vi "FTW-Container-FromVariant.vi"(0 "Variant":variant, 11 "error in":errorcluster) -> (4 "Name":string, 6 "Container":variant, 15 "error out":errorcluster)   [LabVIEW 2015, in "FTW-Container.lvclass"]
uses:
  FTW-Container.lvclass
  <vilib>/Utility/Data Type/NI_Data Type.lvlib
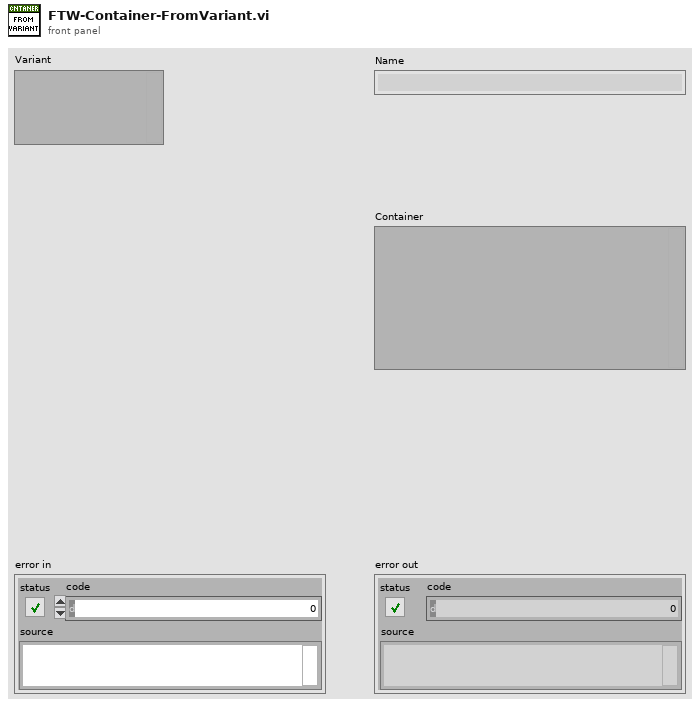
[diagram p1: front panel]
types:
  T1 = typedef "NI_Data Type.lvlib/Data Type.ctl" = enum8{"Invalid Type", "Void", "I8", "I16", "I32", "I64", "U8", "U16", "U32", "U64", "Single Float", "Double Float", "Extended Float", "Single Complex", "Double Complex", "Extended Complex", "Enum U8", "Enum U16", "Enum U32", "Enum U64", "Single Float With Unit", "Double Float With Unit", "Extended Float With Unit", "Single Complex with Unit", "Double Complex with Unit", "Extended Complex with Unit", "Boolean", "String", "Path", "Picture", "Tag", "Array", "Cluster", "Variant", "LV Variant", "Waveform", "Timestamp", "Digital Waveform", "Digital Data", "ExpressData", "Refnum", "External Data", "VI", "Poly VI", "LabVIEW Class Instance", "Fixed Point"}
  T2 = typedef "NI_Data Type.lvlib/Refnum Type.ctl" = enum16{"NotARefnum", "UnknownRefnum", "Generic", "Datalog", "ByteStream", "Device", "Occurence", "TCPNetConnection", "Auto", "Menu", "Imaq", "Hardware", "DataSocket", "Visa", "IVI", "UDPNetConnection", "Notifier", "Queue", "Irda", "EventReg", "DotNet", "UserEvent", "Callback", "UNUSED_EMPTY_POSITION", "BlueToothNetConnection", "LVObjApp", "LVObjVI", "LVObjUnknown", "GenericClass", "UserDefinedRefnumTag", "DataValue", "RT FIFO", "TDMS File"}
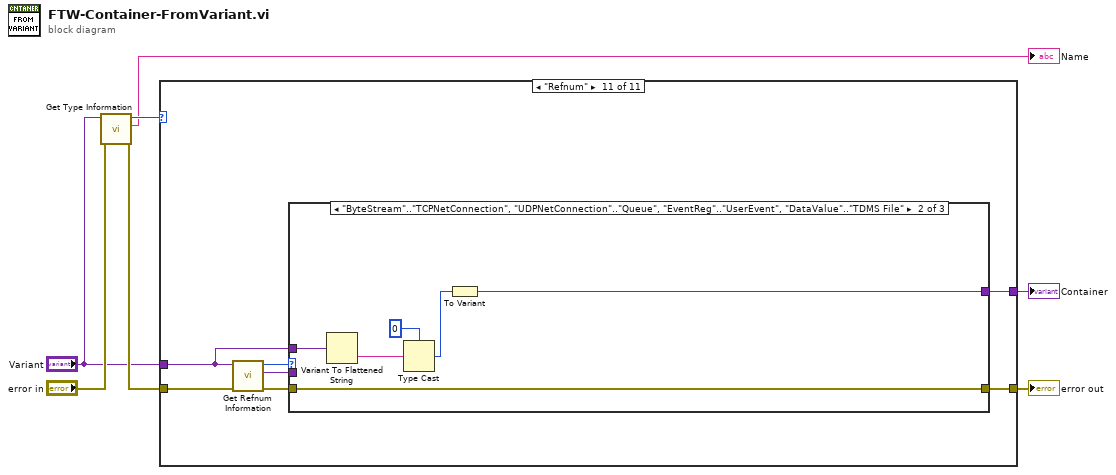
[diagram p0: block diagram]
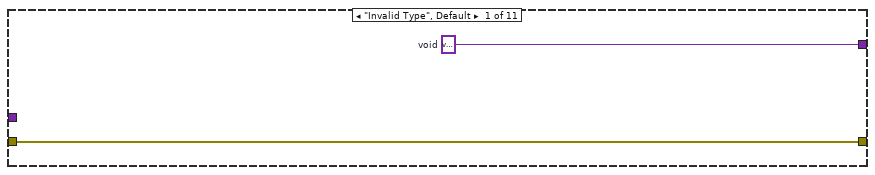
[diagram p2: hidden frame]
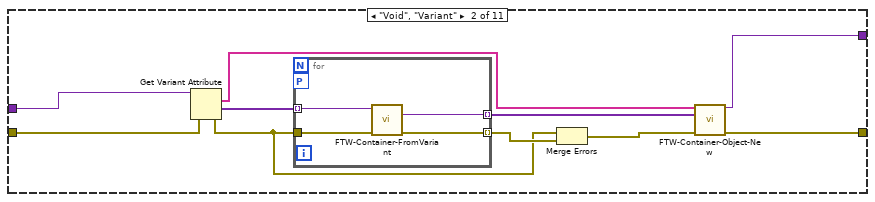
[diagram p3: hidden frame]
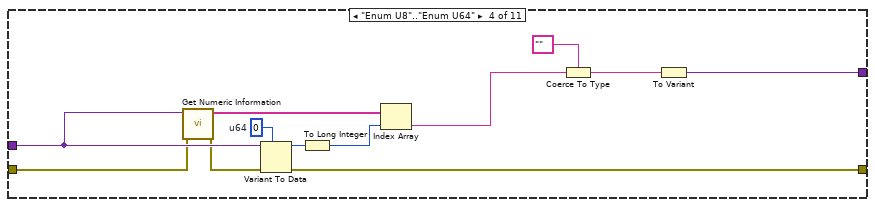
[diagram p5: hidden frame]
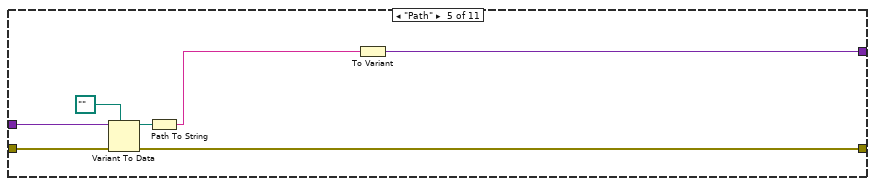
[diagram p6: hidden frame]
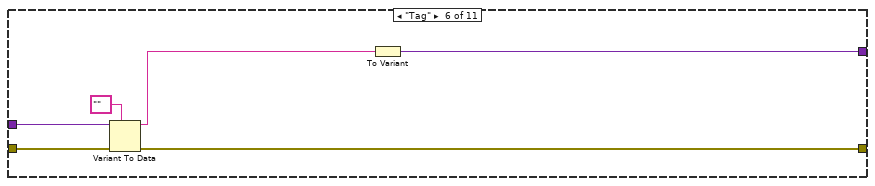
[diagram p7: hidden frame]
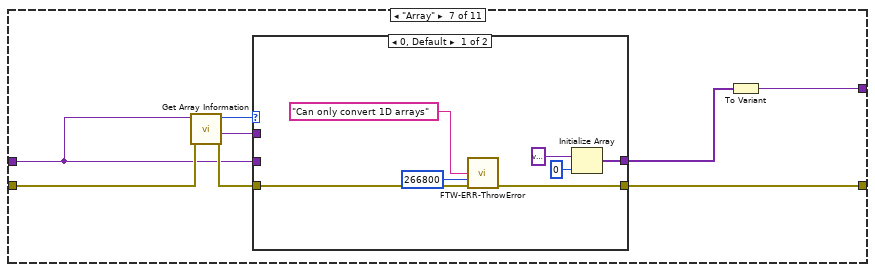
[diagram p8: hidden frame]
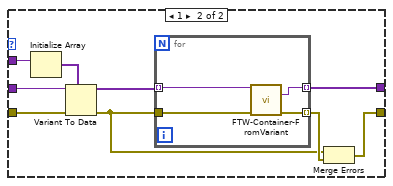
[diagram p9: hidden frame]
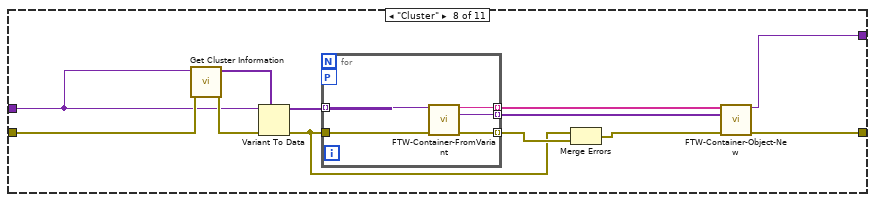
[diagram p10: hidden frame]
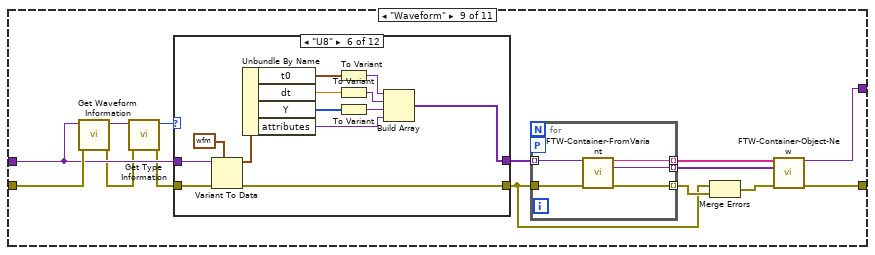
[diagram p11: hidden frame]
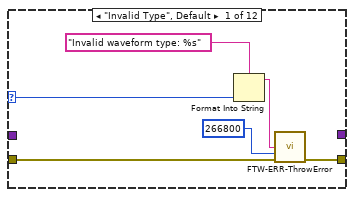
[diagram p12: hidden frame]
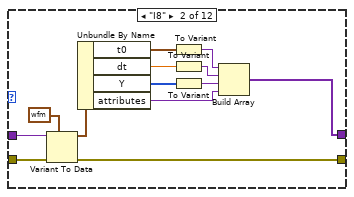
[diagram p13: hidden frame]
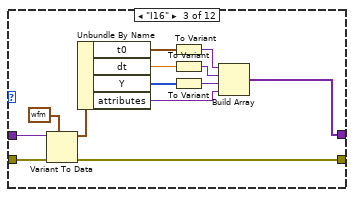
[diagram p14: hidden frame]
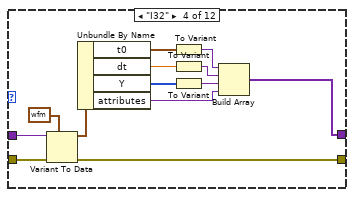
[diagram p15: hidden frame]
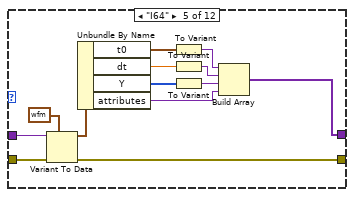
[diagram p16: hidden frame]
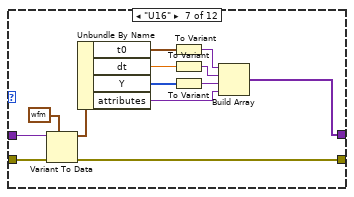
[diagram p17: hidden frame]
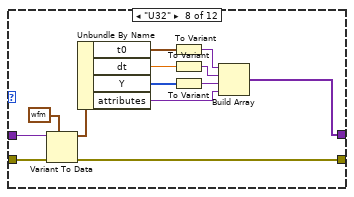
[diagram p18: hidden frame]
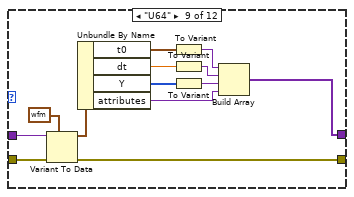
[diagram p19: hidden frame]
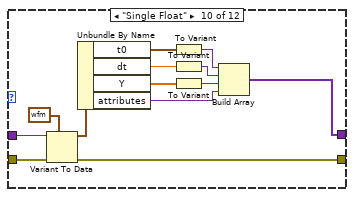
[diagram p20: hidden frame]
diagram:
  n1 = call <vilib>:"Get Type Information.vi"("error in (no error)"="error in", "Variant"="Variant") -> ("error out"=w4:errorcluster, "Name"=→"Name":string, "Type"=w2:T1)  [unwired: 5 in, 2 out]
  n2 = case shown="\"Refnum\"" w2 {
    tunnel: w4 -> [w9 w19 w25 w29 w44 w50 w57 w90 w109 w269 w274]
    tunnel: [w9 w13 w25 w37 w43 w49 w58 w82 w99 w268 w276] -> w6
    tunnel: [w8 w10 w24 w36 w41 w47 w52 w79 w97 w266 w275] -> w5
    tunnel: "Variant" -> [_ w16 w24 w30 w42 w48 w53 w84 w105 w267 w272]
    frame "Invalid Type", Default {
      w8 = variant  # void
    }
    frame "Void", "Variant" {
      n3 = Get Variant Attribute(Variant=w16, error in=w19) -> (names=w11:string[], values=w14:variant[], error out=w15:errorcluster)  [unwired: 2 in, 1 out]
      n4 = for {
        tunnel: w14 -> [w21] mode=indexing
        tunnel: w15 -> [w22]
        tunnel: [w23] -> w18 mode=indexing
        tunnel: [w20] -> w12 mode=indexing
        workers-P: _ -> [_]
        n5 = call "FTW-Container-FromVariant.vi"("Variant"=w21, "error in"=w22) -> ("Container"=w20:variant, "error out"=w23:errorcluster)  [unwired: 11 in, 1 out]
      }
      n6 = Merge Errors(w15, w18) -> (w17:errorcluster)
      n7 = call "FTW-Container-Object-New.vi"("Names"=w11, "Values"=w12, "error in"=w17) -> (4:w10:variant, "error out"=w13:errorcluster)  [unwired: 11 in]
    }
    frame "I8".."Extended Float", "Boolean", "String" {
    }
    frame "Enum U8".."Enum U64" {
      w35 = u64 0  # u64
      n8 = call <vilib>:"Get Numeric Information.vi"("error in (no error)"=w29, "Variant"=w30) -> ("error out"=w28:errorcluster, "Enum Names"=w34:string[])  [unwired: 6 in, 2 out]
      n9 = Variant To Data(error in=w28, type=w35, Variant=w30) -> (data=w33:u64, error out=w37:errorcluster)
      n10 = To Long Integer(number=w33) -> (32bit integer=w32:i32)
      n11 = Index Array(array=w34, index=w32) -> (element=w31:string)
      n12 = Coerce To Type(0:w31, 1:"") -> (2:w27:string)
      n13 = To Variant(anything=w27) -> (Variant=w36:variant)
    }
    frame "Path" {
      n14 = Variant To Data(error in=w44, type=path "", Variant=w42) -> (data=w40:path, error out=w43:errorcluster)
      n15 = Path To String(path=w40) -> (string=w38:string)
      n16 = To Variant(anything=w38) -> (Variant=w41:variant)
    }
    frame "Tag" {
      n17 = Variant To Data(error in=w50, type="", Variant=w48) -> (data=w45:string, error out=w49:errorcluster)
      n18 = To Variant(anything=w45) -> (Variant=w47:variant)
    }
    frame "Array" {
      n19 = call <vilib>:"Get Array Information.vi"("error in (no error)"=w57, "Variant"=w53) -> ("error out"=w56:errorcluster, "Array Element Data Type"=w54:variant, "Number of Dimensions"=w55:i32)  [unwired: 6 in, 1 out]
      n20 = case shown="0, Default" w55 {
        tunnel: [w61 w68] -> w58
        tunnel: w56 -> [w65 w73]
        tunnel: w54 -> [_ w71]
        tunnel: [w64 w66] -> w51
        tunnel: w53 -> [_ w72]
        frame 0, Default {
          n21 = call "FTW-ERR-ThrowError.vi"("Error Message"="Can only convert 1D arrays", "Error Code"=266800, "error in"=w65) -> ("error out"=w61:errorcluster)  [unwired: 12 in]
          n22 = Initialize Array(variant, 0 ("dimension size")) -> (w64:variant[])
        }
        frame 1 {
          n23 = Initialize Array(w71) -> (w70:variant[])  [unwired: 1 in]
          n24 = Variant To Data(error in=w73, type=w70, Variant=w72) -> (data=w69:variant[], error out=w67:errorcluster)
          n25 = for {
            tunnel: w69 -> [w76] mode=indexing
            tunnel: [w75] -> w66 mode=indexing
            tunnel: w67 -> [w77]
            tunnel: [w78] -> w74 mode=indexing
            n26 = call "FTW-Container-FromVariant.vi"("Variant"=w76, "error in"=w77) -> ("Container"=w75:variant, "error out"=w78:errorcluster)  [unwired: 11 in, 1 out]
          }
          n27 = Merge Errors(w67, w74) -> (w68:errorcluster)
        }
      }
      n28 = To Variant(anything=w51) -> (Variant=w52:variant)
    }
    frame "Cluster" {
      n29 = call <vilib>:"Get Cluster Information.vi"("error in (no error)"=w90, "Variant"=w84) -> ("error out"=w87:errorcluster, "Cluster Elements"=w85:variant[])  [unwired: 8 in]
      n30 = Variant To Data(error in=w87, type=w85, Variant=w84) -> (data=w83:variant[], error out=w86:errorcluster)
      n31 = for {
        tunnel: w83 -> [w93] mode=indexing
        tunnel: w86 -> [w95]
        tunnel: [w94] -> w89 mode=indexing
        tunnel: [w92] -> w81 mode=indexing
        tunnel: [w91] -> w80 mode=indexing
        workers-P: _ -> [_]
        n32 = call "FTW-Container-FromVariant.vi"("Variant"=w93, "error in"=w95) -> ("Name"=w92:string, "Container"=w91:variant, "error out"=w94:errorcluster)  [unwired: 11 in]
      }
      n33 = Merge Errors(w86, w89) -> (w88:errorcluster)
      n34 = call "FTW-Container-Object-New.vi"("Names"=w81, "Values"=w80, "error in"=w88) -> (4:w79:variant, "error out"=w82:errorcluster)  [unwired: 11 in]
    }
    frame "Waveform" {
      n35 = call <vilib>:"Get Waveform Information.vi"("error in (no error)"=w109, "Variant"=w105) -> ("error out"=w102:errorcluster, "Y Array Type"=w103:variant)  [unwired: 8 in]
      n36 = call <vilib>:"Get Type Information.vi"("error in (no error)"=w102, "Variant"=w103) -> ("error out"=w101:errorcluster, "Type"=w100:T1)  [unwired: 5 in, 3 out]
      n37 = case shown="\"U8\"" w100 {
        selector: w100 -> [w111 _ _ _ _ _ _ _ _ _ _ _]
        tunnel: [w114 w117 w130 w143 w156 w169 w182 w195 w208 w221 w234 w247] -> w106
        tunnel: w105 -> [_ w120 w133 w146 w159 w172 w185 w198 w211 w224 w237 w250]
        tunnel: [_ w128 w141 w154 w167 w180 w193 w206 w219 w232 w245 w258] -> w104
        tunnel: w101 -> [w115 w124 w137 w150 w163 w176 w189 w202 w215 w228 w241 w254]
        frame "Invalid Type", Default {
          n38 = Format Into String(format string="Invalid waveform type: %s" ("Error Message"), w111) -> (resulting string=w110:string)  [unwired: 2 in, 1 out]
          n39 = call "FTW-ERR-ThrowError.vi"("Error Message"=w110, "Error Code"=266800, "error in"=w115) -> ("error out"=w114:errorcluster)  [unwired: 12 in]
        }
        frame "I8" {
          n40 = Variant To Data(error in=w124, type=waveform(i8) {"t0"=timestamp(0 s since 1904-01-01), "dt"=1.0, "Y"=[]} ("Waveform"), Variant=w120) -> (data=w118:waveform(i8), error out=w117:errorcluster)
          n41 = Unbundle By Name(w118) -> ("t0"=w123:timestamp, "dt"=w122:dbl, "Y"=w121:i8[], "attributes"=w116:variant)
          n42 = To Variant(anything=w123) -> (Variant=w127:variant)
          n43 = To Variant(anything=w122) -> (Variant=w126:variant)
          n44 = To Variant(anything=w121) -> (Variant=w125:variant)
          n45 = Build Array(w127, w126, w125, w116) -> (w128:variant[])
        }
        frame "I16" {
          n46 = Variant To Data(error in=w137, type=waveform(i16) {"t0"=timestamp(0 s since 1904-01-01), "dt"=1.0, "Y"=[]} ("Waveform"), Variant=w133) -> (data=w131:waveform(i16), error out=w130:errorcluster)
          n47 = Unbundle By Name(w131) -> ("t0"=w136:timestamp, "dt"=w135:dbl, "Y"=w134:i16[], "attributes"=w129:variant)
          n48 = To Variant(anything=w136) -> (Variant=w140:variant)
          n49 = To Variant(anything=w135) -> (Variant=w139:variant)
          n50 = To Variant(anything=w134) -> (Variant=w138:variant)
          n51 = Build Array(w140, w139, w138, w129) -> (w141:variant[])
        }
        frame "I32" {
          n52 = Variant To Data(error in=w150, type=waveform(i32) {"t0"=timestamp(0 s since 1904-01-01), "dt"=1.0, "Y"=[]} ("Waveform"), Variant=w146) -> (data=w144:waveform(i32), error out=w143:errorcluster)
          n53 = Unbundle By Name(w144) -> ("t0"=w149:timestamp, "dt"=w148:dbl, "Y"=w147:i32[], "attributes"=w142:variant)
          n54 = To Variant(anything=w149) -> (Variant=w153:variant)
          n55 = To Variant(anything=w148) -> (Variant=w152:variant)
          n56 = To Variant(anything=w147) -> (Variant=w151:variant)
          n57 = Build Array(w153, w152, w151, w142) -> (w154:variant[])
        }
        frame "I64" {
          n58 = Variant To Data(error in=w163, type=waveform(i64) {"t0"=timestamp(0 s since 1904-01-01), "dt"=1.0, "Y"=[]} ("Waveform"), Variant=w159) -> (data=w157:waveform(i64), error out=w156:errorcluster)
          n59 = Unbundle By Name(w157) -> ("t0"=w162:timestamp, "dt"=w161:dbl, "Y"=w160:i64[], "attributes"=w155:variant)
          n60 = To Variant(anything=w162) -> (Variant=w166:variant)
          n61 = To Variant(anything=w161) -> (Variant=w165:variant)
          n62 = To Variant(anything=w160) -> (Variant=w164:variant)
          n63 = Build Array(w166, w165, w164, w155) -> (w167:variant[])
        }
        frame "U8" {
          n64 = Variant To Data(error in=w176, type=waveform(u8) {"t0"=timestamp(0 s since 1904-01-01), "dt"=1.0, "Y"=[]} ("Waveform"), Variant=w172) -> (data=w170:waveform(u8), error out=w169:errorcluster)
          n65 = Unbundle By Name(w170) -> ("t0"=w175:timestamp, "dt"=w174:dbl, "Y"=w173:u8[], "attributes"=w168:variant)
          n66 = To Variant(anything=w175) -> (Variant=w179:variant)
          n67 = To Variant(anything=w174) -> (Variant=w178:variant)
          n68 = To Variant(anything=w173) -> (Variant=w177:variant)
          n69 = Build Array(w179, w178, w177, w168) -> (w180:variant[])
        }
        frame "U16" {
          n70 = Variant To Data(error in=w189, type=waveform(u16) {"t0"=timestamp(0 s since 1904-01-01), "dt"=1.0, "Y"=[]} ("Waveform"), Variant=w185) -> (data=w183:waveform(u16), error out=w182:errorcluster)
          n71 = Unbundle By Name(w183) -> ("t0"=w188:timestamp, "dt"=w187:dbl, "Y"=w186:u16[], "attributes"=w181:variant)
          n72 = To Variant(anything=w188) -> (Variant=w192:variant)
          n73 = To Variant(anything=w187) -> (Variant=w191:variant)
          n74 = To Variant(anything=w186) -> (Variant=w190:variant)
          n75 = Build Array(w192, w191, w190, w181) -> (w193:variant[])
        }
        frame "U32" {
          n76 = Variant To Data(error in=w202, type=waveform(u32) {"t0"=timestamp(0 s since 1904-01-01), "dt"=1.0, "Y"=[]} ("Waveform"), Variant=w198) -> (data=w196:waveform(u32), error out=w195:errorcluster)
          n77 = Unbundle By Name(w196) -> ("t0"=w201:timestamp, "dt"=w200:dbl, "Y"=w199:u32[], "attributes"=w194:variant)
          n78 = To Variant(anything=w201) -> (Variant=w205:variant)
          n79 = To Variant(anything=w200) -> (Variant=w204:variant)
          n80 = To Variant(anything=w199) -> (Variant=w203:variant)
          n81 = Build Array(w205, w204, w203, w194) -> (w206:variant[])
        }
        frame "U64" {
          n82 = Variant To Data(error in=w215, type=waveform(u64) {"t0"=timestamp(0 s since 1904-01-01), "dt"=1.0, "Y"=[]} ("Waveform"), Variant=w211) -> (data=w209:waveform(u64), error out=w208:errorcluster)
          n83 = Unbundle By Name(w209) -> ("t0"=w214:timestamp, "dt"=w213:dbl, "Y"=w212:u64[], "attributes"=w207:variant)
          n84 = To Variant(anything=w214) -> (Variant=w218:variant)
          n85 = To Variant(anything=w213) -> (Variant=w217:variant)
          n86 = To Variant(anything=w212) -> (Variant=w216:variant)
          n87 = Build Array(w218, w217, w216, w207) -> (w219:variant[])
        }
        frame "Single Float" {
          n88 = Variant To Data(error in=w228, type=waveform(sgl) {"t0"=timestamp(0 s since 1904-01-01), "dt"=1.0, "Y"=[]} ("Waveform"), Variant=w224) -> (data=w222:waveform(sgl), error out=w221:errorcluster)
          n89 = Unbundle By Name(w222) -> ("t0"=w227:timestamp, "dt"=w226:dbl, "Y"=w225:sgl[], "attributes"=w220:variant)
          n90 = To Variant(anything=w227) -> (Variant=w231:variant)
          n91 = To Variant(anything=w226) -> (Variant=w230:variant)
          n92 = To Variant(anything=w225) -> (Variant=w229:variant)
          n93 = Build Array(w231, w230, w229, w220) -> (w232:variant[])
        }
        frame "Double Float" {
          n94 = Variant To Data(error in=w241, type=waveform(dbl) {"t0"=timestamp(0 s since 1904-01-01), "dt"=1.0, "Y"=[]} ("Waveform"), Variant=w237) -> (data=w235:waveform(dbl), error out=w234:errorcluster)
          n95 = Unbundle By Name(w235) -> ("t0"=w240:timestamp, "dt"=w239:dbl, "Y"=w238:dbl[], "attributes"=w233:variant)
          n96 = To Variant(anything=w240) -> (Variant=w244:variant)
          n97 = To Variant(anything=w239) -> (Variant=w243:variant)
          n98 = To Variant(anything=w238) -> (Variant=w242:variant)
          n99 = Build Array(w244, w243, w242, w233) -> (w245:variant[])
        }
        frame "Extended Float" {
          n100 = Variant To Data(error in=w254, type=waveform(ext) {"t0"=timestamp(0 s since 1904-01-01), "dt"=1.0, "Y"=[]} ("Waveform"), Variant=w250) -> (data=w248:waveform(ext), error out=w247:errorcluster)
          n101 = Unbundle By Name(w248) -> ("t0"=w253:timestamp, "dt"=w252:dbl, "Y"=w251:ext[], "attributes"=w246:variant)
          n102 = To Variant(anything=w253) -> (Variant=w257:variant)
          n103 = To Variant(anything=w252) -> (Variant=w256:variant)
          n104 = To Variant(anything=w251) -> (Variant=w255:variant)
          n105 = Build Array(w257, w256, w255, w246) -> (w258:variant[])
        }
      }
      n106 = for {
        tunnel: w104 -> [w261] mode=indexing
        tunnel: w106 -> [w262]
        tunnel: [w263] -> w108 mode=indexing
        workers-P: _ -> [_]
        tunnel: [w260] -> w96 mode=indexing
        tunnel: [w259] -> w98 mode=indexing
        n107 = call "FTW-Container-FromVariant.vi"("Variant"=w261, "error in"=w262) -> ("Name"=w259:string, "Container"=w260:variant, "error out"=w263:errorcluster)  [unwired: 11 in]
      }
      n108 = Merge Errors(w106, w108) -> (w107:errorcluster)
      n109 = call "FTW-Container-Object-New.vi"("Names"=w98, "Values"=w96, "error in"=w107) -> (4:w97:variant, "error out"=w99:errorcluster)  [unwired: 11 in]
    }
    frame "Timestamp" {
      n110 = Variant To Data(error in=w269, type=timestamp(0 s since 1904-01-01), Variant=w267) -> (data=w264:timestamp, error out=w268:errorcluster)
      n111 = To Variant(anything=w264) -> (Variant=w266:variant)
    }
    frame "Refnum" {
      n112 = call <vilib>:"Get Refnum Information.vi"("error in (no error)"=w274, "Variant"=w272) -> ("error out"=w273:errorcluster, "Strict Type"=w270:variant, "Reference Type"=w271:T2)  [unwired: 6 in, 1 out]
      n113 = case shown="\"ByteStream\"..\"TCPNetConnection\", \"UDPNetConnection\"..\"Queue\", \"EventReg\"..\"UserEvent\", \"DataValue\"..\"TDMS File\"" w271 {
        tunnel: [w278 w281 w290] -> w276
        tunnel: [variant ("empty string") w284 w289] -> w275
        tunnel: w273 -> [w278 w281 w286]
        tunnel: w272 -> [_ w280 w285]
        tunnel: w270 -> [_ _ _]
        frame "NotARefnum", Default {
        }
        frame "ByteStream".."TCPNetConnection", "UDPNetConnection".."Queue", "EventReg".."UserEvent", "DataValue".."TDMS File" {
          n114 = Variant To Flattened String(Variant=w280) -> (data string=w279:string)  [unwired: 1 out]
          n115 = Type Cast(type=u32 0, x=w279) -> (*(type *) &x=w282:u32)
          n116 = To Variant(anything=w282) -> (Variant=w284:variant)
        }
        frame "Visa", "UserDefinedRefnumTag" {
          n117 = Variant To Data(error in=w286, type="", Variant=w285) -> (data=w287:string, error out=w290:errorcluster)
          n118 = To Variant(anything=w287) -> (Variant=w289:variant)
        }
      }
    }
  }
  "error out" <- w6
  "Container" <- w5
